vi "Log Pattern.vi"(0 "P1 CH0, V":dbl=3.3000000000000003 caption="voltage level" min=0.0 max=6.0 format="%_6p", 1 "P1 CH0_cur, A":dbl=8.200132019086688e-05 caption="measurement" format="%_6g", 2 "P1 CH0_counter":u32 caption="VCC_counter", 3 "SEL Mark In Log":string, 4 "P CH_warning":bool, 5 "P1 CH0 Used":bool, 8 "Significant Digits":i16) -> (16 "Log Pattern String":string)   [LabVIEW 2018]
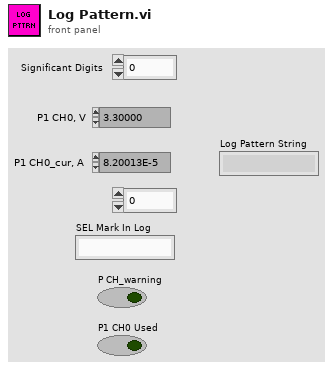
[diagram p1: front panel]
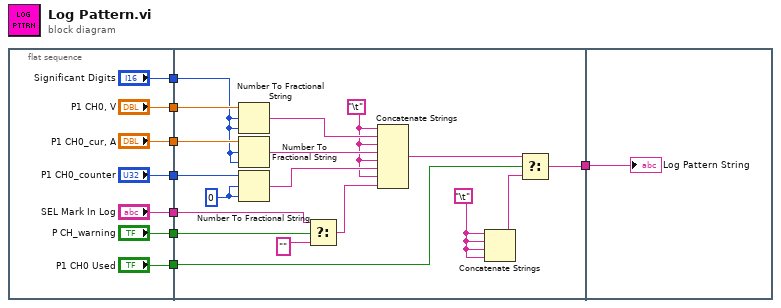
[diagram p0: block diagram]
diagram:
  n1 = flat-sequence {
    tunnel: ["P1 CH0, V"] -> w8
    tunnel: ["P1 CH0_cur, A"] -> w7
    tunnel: ["P1 CH0_counter"] -> w6
    tunnel: ["P CH_warning"] -> w5
    tunnel: ["P1 CH0 Used"] -> w4
    tunnel: ["Significant Digits"] -> w3
    tunnel: ["SEL Mark In Log"] -> w1
    tunnel: w8 -> [w32]
    tunnel: w7 -> [w31]
    tunnel: w6 -> [w29]
    tunnel: w5 -> [w20]
    tunnel: w4 -> [w19]
    tunnel: w3 -> [w18]
    tunnel: [w17] -> w2
    tunnel: w1 -> [w16]
    tunnel: w2 -> [w34]
    frame #0 {
    }
    frame #1 {
      w23 = "\t"
      w21 = "\t"
      w30 = 0
      n2 = Number To Fractional String(number=w32, width (-)=w18, precision (6)=w18) -> (F-format string=w28:string)  [unwired: 1 in]
      n3 = Number To Fractional String(number=w31, width (-)=w18, precision (6)=w18) -> (F-format string=w27:string)  [unwired: 1 in]
      n4 = Number To Fractional String(number=w29, width (-)=w30, precision (6)=w30) -> (F-format string=w26:string)  [unwired: 1 in]
      n5 = Select(t=w16, s=w20, f="") -> (s? t:f=w25:string)
      n6 = Concatenate Strings(w21, w28, w21, w27, w21, w26, w21, w25) -> (w24:string)
      n7 = Concatenate Strings(w23, w23, w23, w23) -> (w22:string)
      n8 = Select(t=w24, s=w19, f=w22) -> (s? t:f=w17:string)
    }
    frame #2 {
      "Log Pattern String" <- w34
    }
  }
